vi "TEMP VISA CLOSE TEST.vi"() -> ()   [LabVIEW 2017]
panel:
  out "Cluster OUT":T1
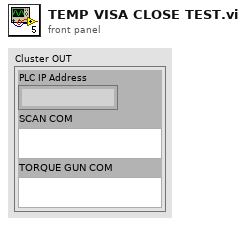
[diagram p1: front panel]
types:
  T1 = cluster{"PLC IP Address":string, "SCAN COM":refnum<visa-resource-name>, "TORQUE GUN COM":refnum<visa-resource-name>}
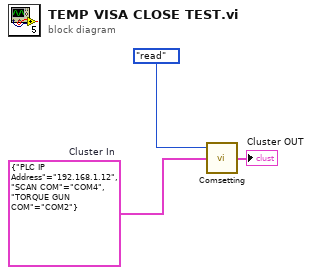
[diagram p0: block diagram]
diagram:
  w1 = T1 {"PLC IP Address"="192.168.1.12", "SCAN COM"="COM4", "TORQUE GUN COM"="COM2"}  # Cluster In
  n1 = call "Comsetting.vi"("Cluster In"=w1, "Enum"=enum16{"read", "write"}."read") -> ("Cluster OUT"=→"Cluster OUT":T1)  [unwired: 1 in, 2 out]
